vi "Is-Axis-Moving.vi"(5 "error in":errorcluster) -> (0 "error out":errorcluster, 1 "Z":bool, 2 "Y":bool, 3 "X":bool)   [LabVIEW 2017]
uses:
  ICNC/ICNC2.lvlib
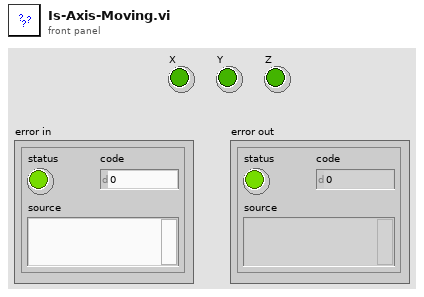
[diagram p1: front panel]
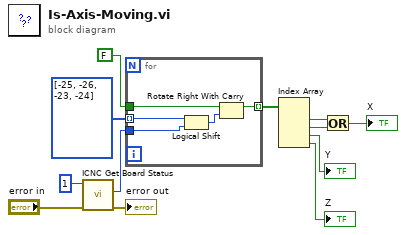
[diagram p0: block diagram]
diagram:
  n1 = call <menus>:"ICNC Get Board Status.vi"("error in (no error)"="error in", "StatusType"=u32 1 ("ParameterID")) -> ("error out"=→"error out":errorcluster, "Status out"=w9:u32)  [unwired: 7 in, 1 out]
  n2 = for {
    tunnel: i16[] [-25, -26, -23, -24] -> [w13] mode=indexing
    tunnel: w9 -> [w17]
    tunnel: [w15] -> w7 mode=indexing
    tunnel: FALSE ("carry") -> [w14]
    n3 = Logical Shift(y=w13, x=w17) -> (x << y=w16:u32)
    n4 = Rotate Right With Carry(2:w16, 3:w14) -> (1:w15:bool)  [unwired: 1 out]
  }
  n5 = Index Array(array=w7) -> (element #1=w6:bool, element #2=w5:bool, element #3=→"Y":bool, element #4=→"Z":bool)  [unwired: 4 in]
  n6 = Or(x=w6, y=w5) -> (x .or. y?=→"X":bool)
